vi "Set Controls.vi"(4 "Ignore Non-existent Controls":bool, 6 "VI Control Values":refnum<class "tBSONDocument.lvclass">, 7 "Project Path":string, 8 "error in (no error)":errorcluster, 9 "VI Path":string, 10 "Target Name":string, 11 "tWorkerCommandRunner in":refnum<class "tWorkerCommandRunner.lvclass">) -> (0 "error out":errorcluster, 3 "tWorkerCommandRunner out":refnum<class "tWorkerCommandRunner.lvclass">)   [LabVIEW 2014, in "tWorkerCommandRunner.lvlib" / "tWorkerCommandRunner.lvclass"]
uses:
  tWorkerCommandRunner.lvclass
  BSON/tBSONDocument/tBSONDocument.lvclass
  <vilib>/ActorFramework/Actor/Actor.lvclass/Actor.ctl
  BSON/tBSONElement/tBSONElement.lvclass
  tWorkerTCPConnection/msgs/Return Run VI State Msg/Return Run VI State Msg.lvclass
  <vilib>/ActorFramework/Actor/Actor.lvclass
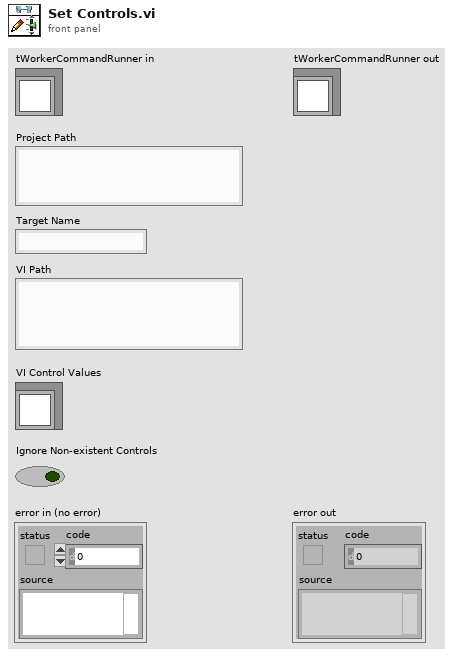
[diagram p1: front panel]
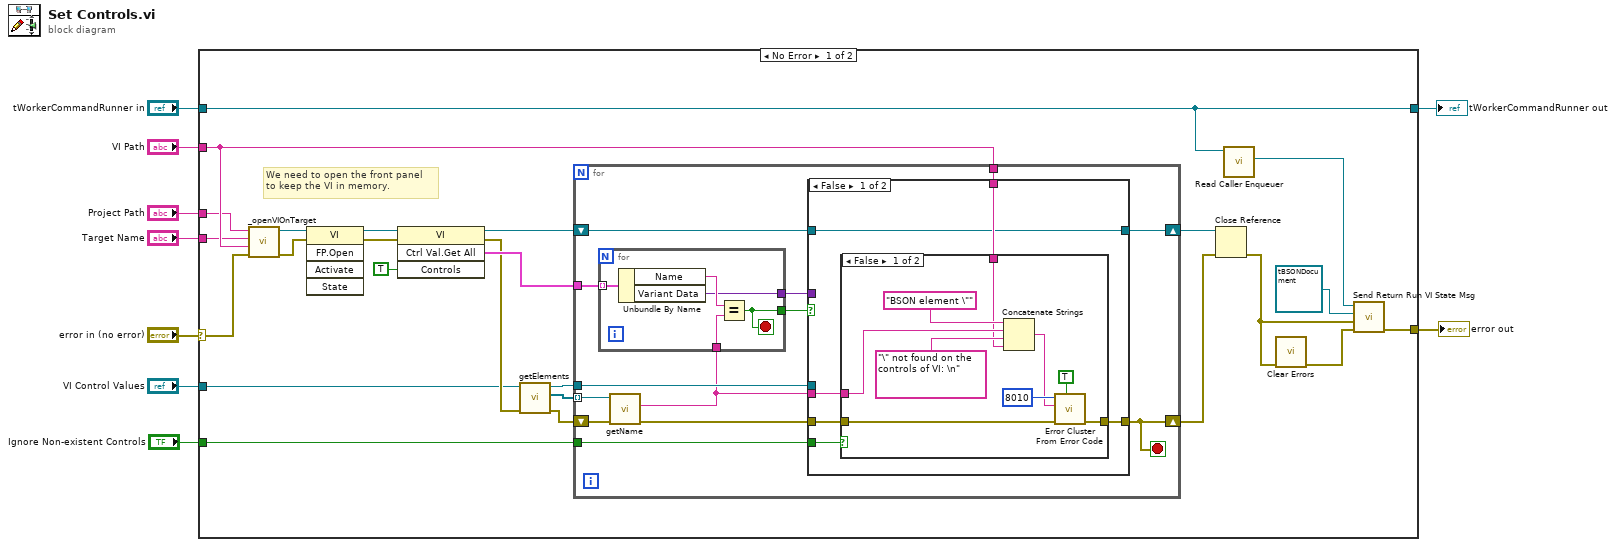
[diagram p0: block diagram]
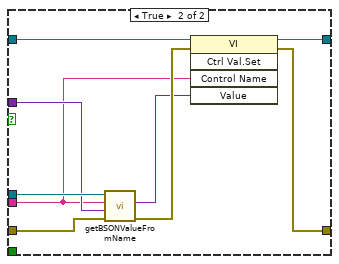
[diagram p3: hidden frame]
diagram:
  n1 = case shown="No Error" "error in (no error)" {
    selector: "error in (no error)" -> [w23 w79]
    tunnel: [w16 w79] -> w8
    tunnel: [w19 w78] -> w6
    tunnel: "tWorkerCommandRunner in" -> [w19 w78]
    tunnel: "VI Control Values" -> [w27 _]
    tunnel: "VI Path" -> [w26 _]
    tunnel: "Project Path" -> [w25 _]
    tunnel: "Target Name" -> [w24 _]
    tunnel: "Ignore Non-existent Controls" -> [w14 _]
    frame No Error {
      # "We need to open the front panel\nto keep the VI in memory."
      n2 = call "_openVIOnTarget.vi"("error in (no error)"=w23, "VI Path"=w26, "Target Name"=w24, "Project Path"=w25) -> ("error out"=w12:errorcluster, "VI Reference"=w13:refnum<vi>)  [unwired: 6 in]
      n3 = invoke class="VI" method="FP.Open"(reference=w13, error in=w12) -> (reference out=w11:refnum<vi>, error out=w10:errorcluster)  [unwired: 3 in, 3 out]
      n4 = invoke class="VI" method="Ctrl Val.Get All"(reference=w11, error in=w10, "Controls"=TRUE) -> (reference out=w34:refnum<vi>, error out=w29:errorcluster, "Get All Control Values Variant"=w32:cluster{"Name":string, "Variant Data":variant}[])  [unwired: 1 in, 1 out]
      n5 = call "getElements.vi"("error in (no error)"=w29, "tBSONDocument in"=w27) -> ("error out"=w30:errorcluster, "Elements"=w31:refnum<class "tBSONElement.lvclass">[], "tBSONDocument out"=w33:refnum<class "tBSONDocument.lvclass">)  [unwired: 7 in]
      n6 = for {
        tunnel: w31 -> [w47] mode=indexing
        shift-right: [w37] -> w17
        shift-left: w30 -> [w46]
        tunnel: w32 -> [w45]
        tunnel: w33 -> [w43]
        shift-right: [w38] -> w18
        shift-left: w34 -> [w41]
        tunnel: w26 -> [w39]
        tunnel: w14 -> [w35]
        stop <- w37 stop-if-true
        n7 = call "getName.vi"("error in (no error)"=w46, "tBSONElement in"=w47) -> ("error out"=w44:errorcluster, "Name"=w40:string)  [unwired: 7 in, 1 out]
        n8 = for {
          tunnel: w45 -> [w77] mode=indexing
          tunnel: w40 -> [w75]
          tunnel: [w74] -> w42
          tunnel: [w73] -> w36
          stop <- w73 stop-if-true
          n9 = Unbundle By Name(w77) -> ("Name"=w76:string, "Variant Data"=w74:variant)
          n10 = Equal?(x=w76, y=w75) -> (x = y?=w73:bool)
        }
        n11 = case shown="False" w36 {
          tunnel: w44 -> [w53 w71]
          tunnel: w43 -> [_ w72]
          tunnel: w42 -> [_ w70]
          tunnel: w41 -> [w49 w69]
          tunnel: w40 -> [w51 w67]
          tunnel: [w52 w64] -> w37
          tunnel: w39 -> [w50 _]
          tunnel: [w49 w65] -> w38
          tunnel: w35 -> [w48 _]
          frame False {
            n12 = case shown="False" w48 {
              tunnel: w53 -> [w62 w63]
              tunnel: [w59 w63] -> w52
              tunnel: w51 -> [w56 _]
              tunnel: w50 -> [w54 _]
              frame False {
                n13 = Concatenate Strings("BSON element \"" ("string"), w56, "\" not found on the controls of VI: \n" ("string"), w54) -> (w57:string)
                n14 = call <vilib>:"Error Cluster From Error Code.vi"("show call chain? (False)"=TRUE, "error in (no error)"=w62, "error message (\"\")"=w57, "error code (0)"=8010) -> ("error out"=w59:errorcluster)  [unwired: 5 in]
              }
              frame True {
                # "Couldn't find control, but the\nignore flag is True."
              }
            }
          }
          frame True {
            n15 = call "getBSONValueFromName.vi"("error in (no error)"=w71, "Cluster Type (optional)"=w70, "Element Name"=w67, "tBSONDocument in"=w72) -> ("error out"=w68:errorcluster, "Variant"=w66:variant)  [unwired: 5 in, 1 out]
            n16 = invoke class="VI" method="Ctrl Val.Set"(reference=w69, error in=w68, "Control Name"=w67, "Value"=w66) -> (reference out=w65:refnum<vi>, error out=w64:errorcluster)  [unwired: 1 in, 3 out]
          }
        }
      }
      n17 = Close Reference(reference=w18, error in (no error)=w17) -> (error out=w21:errorcluster)
      n18 = call <vilib>:"Read Caller Enqueuer.vi"("Actor"=w19) -> ("Caller Enqueuer"=w22:refnum<class "Message Enqueuer.lvclass">)  [unwired: 10 in]
      n19 = call <vilib>:"Clear Errors.vi"("error in (no error)"=w21) -> ("error out"=w20:errorcluster)  [unwired: 5 in, 1 out]
      n20 = call "Send Return Run VI State Msg.vi"("error in (no error)"=w20, "Error From Run VI"=w21, "Indicators"=refnum<class "tBSONDocument.lvclass"> refnum, "Message Enqueuer"=w22) -> ("error out"=w16:errorcluster)  [unwired: 6 in, 1 out]
    }
    frame Error {
    }
  }
  "error out" <- w8
  "tWorkerCommandRunner out" <- w6
